vi "SetAveraging.vi"(3 "Averages":i32=1, 4 "Device":u8=1, 5 "Serial port":refnum<visa-resource-name>) -> (1 "Device out":u8=1, 2 "Serial port out":refnum<visa-resource-name>)   [LabVIEW 2021]
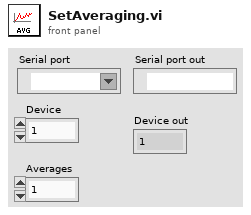
[diagram p1: front panel]
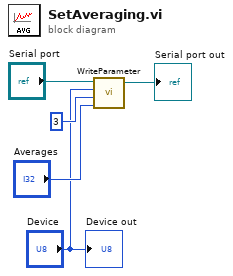
[diagram p0: block diagram]
diagram:
  n1 = call "WriteParameter.vi"("Value"="Averages", "Address"=u32 3, "Device"="Device", "Serial port"="Serial port") -> ("Serial port out"=→"Serial port out":refnum<visa-resource-name>)  [unwired: 2 in]
  "Device out" <- "Device"
